vi "Scroll Image.vi"(7 "Reset? (F)":bool, 9 "Height":i32, 10 "Width":i32, 11 "Image Array In":i32[](array[numeric])) -> (3 "Image Array Out":i32[](array[numeric]))   [LabVIEW 2019]
doc: "Scrolls the input image 1 line vertically every call. The image stops scrolling when it is fully visible.\n\nThe scroll can be restarted by setting the Reset? input to true."
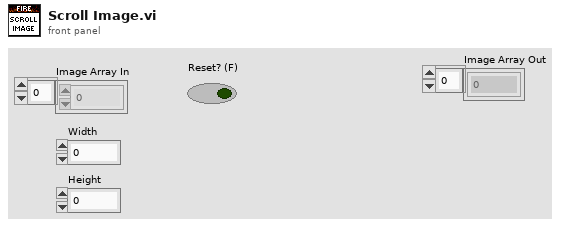
[diagram p1: front panel]
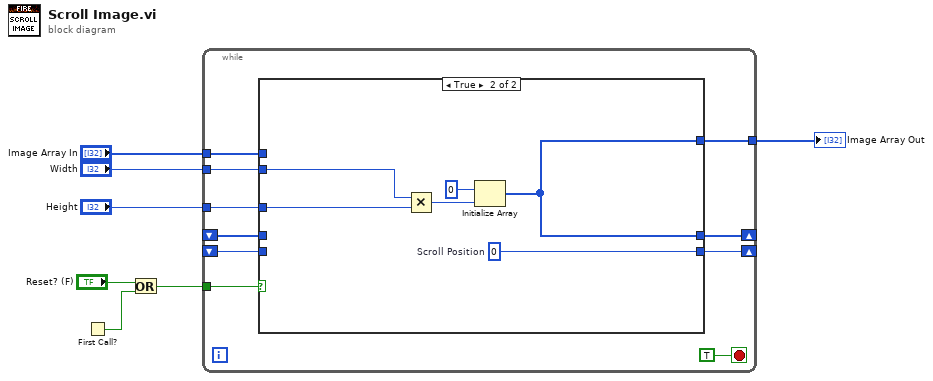
[diagram p0: block diagram]
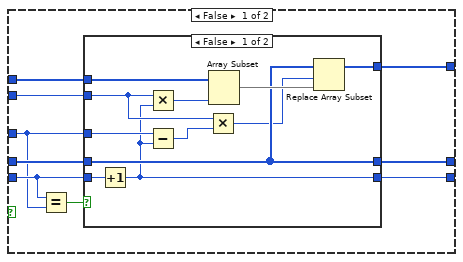
[diagram p2: hidden frame]
diagram:
  n1 = First Call?() -> (First Call?: T/F=w6:bool)
  n2 = Or(x="Reset? (F)", y=w6) -> (x .or. y?=w4:bool)
  n3 = while {
    tunnel: "Image Array In" -> [w10]
    tunnel: w4 -> [w17]
    tunnel: "Width" -> [w16]
    tunnel: "Height" -> [w15]
    shift-right: [w14] -> _
    shift-left: _ -> [w13]
    shift-right: [w12] -> _
    shift-left: _ -> [w11]
    tunnel: [w9] -> w1
    stop <- TRUE stop-if-true
    n4 = case shown="True" w17 {
      tunnel: w16 -> [w22 w46]
      tunnel: w15 -> [w18 w45]
      tunnel: [w19 w41] -> w14
      tunnel: w13 -> [w25 _]
      tunnel: [w23 w42] -> w12
      tunnel: w11 -> [w21 _]
      tunnel: w10 -> [w26 _]
      tunnel: [w24 w41] -> w9
      frame False {
        n5 = Equal?(x=w21, y=w18) -> (x = y?=w20:bool)
        n6 = case shown="False" w20 {
          tunnel: w26 -> [w37 w40]
          tunnel: w25 -> [w32 w39]
          tunnel: [w36 w40] -> w24
          tunnel: w21 -> [w35 w38]
          tunnel: [w27 w38] -> w23
          tunnel: w22 -> [w30 _]
          tunnel: [w32 w39] -> w19
          tunnel: w18 -> [w31 _]
          frame False {
            n7 = Increment(x=w35) -> (x+1=w27:i32)
            n8 = Multiply(x=w30, y=w27) -> (x*y=w33:i32)
            n9 = Subtract(x=w31, y=w27) -> (x-y=w29:i32)
            n10 = Multiply(x=w30, y=w29) -> (x*y=w28:i32)
            n11 = Array Subset(array=w37, length=w33) -> (w34:i32[])  [unwired: 1 in]
            n12 = Replace Array Subset(array=w32, new element=w34, index=w28) -> (w36:i32[])
          }
          frame True {
          }
        }
      }
      frame True {
        w42 = 0  # Scroll Position
        n13 = Multiply(x=w46, y=w45) -> (x*y=w44:i32)
        n14 = Initialize Array(0 ("element"), w44) -> (w41:i32[])
      }
    }
  }
  "Image Array Out" <- w1
